vi "TEST - Current VIs Parents Ref.vi"(8 "error in (no error)":errorcluster) -> (0 "error out":errorcluster, 2 "pass":bool)   [LabVIEW 2009]
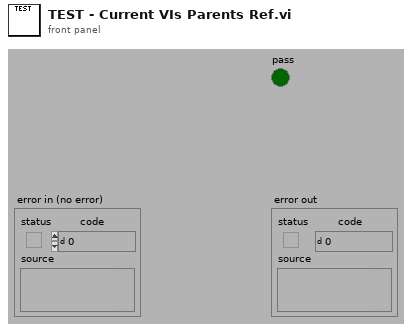
[diagram p1: front panel]
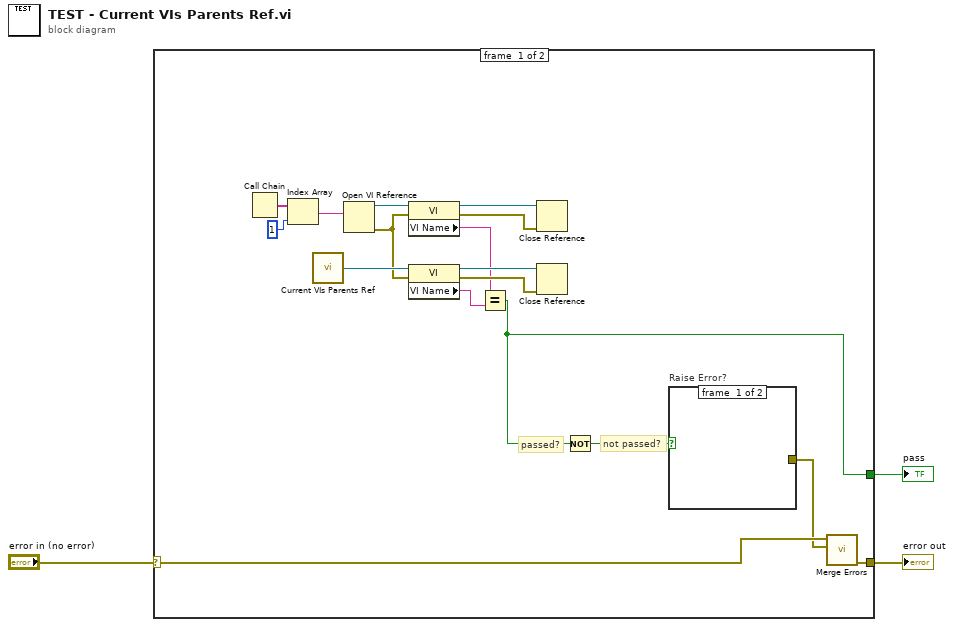
[diagram p0: block diagram]
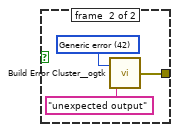
[diagram p2: hidden frame]
diagram:
  n1 = case shown="No Error" "error in (no error)" {
    selector: "error in (no error)" -> [w20 w24]
    tunnel: [w4 _] -> w3
    tunnel: [w19 w24] -> w1
    frame #0 {
      # "not passed?"
      # "passed?"
      n2 = Call Chain() -> (call chain=w16:string[])
      n3 = Index Array(array=w16, index=1 ("Index")) -> (element=w14:string)
      n4 = call "Current VIs Parents Ref.vi"() -> ("Calling VI's reference"=w8:refnum<vi>)  [unwired: 2 in]
      n5 = Open VI Reference(vi path=w14) -> (vi reference=w13:refnum<vi>, error out=w5:errorcluster)  [unwired: 5 in]
      n6 = property class="VI"(reference=w13, error in=w5) -> (reference out=w12:refnum<vi>, error out=w11:errorcluster, "VI Name"=w6:string)
      n7 = property class="VI"(reference=w8, error in=w5) -> (reference out=w9:refnum<vi>, error out=w10:errorcluster, "VI Name"=w7:string)
      n8 = Equal?(x=w6, y=w7) -> (x = y?=w4:bool)
      n9 = Close Reference(reference=w12, error in (no error)=w11) -> ()  [unwired: 1 out]
      n10 = Close Reference(reference=w9, error in (no error)=w10) -> ()  [unwired: 1 out]
      n11 = Not(x=w4) -> (.not. x?=w17:bool)
      n12 = case "Raise Error?" shown="True" w17 {
        tunnel: [_ w21] -> w18
        frame #0 {
        }
        frame #1 {
          w22 = 42 items=["No error", "Argument error", "Memory is full", "Out of zone", "End of file", "File already open", "Generic file I/O error", "File not found", "File permission error", "Disk is full", "Duplicate path", "Too many files open", "System feature not enabled", "Resource file not found", "Cannot add resource", "Resource not found", "Image not found", "Image memory error", "Pen does not exist", "Config type invalid", "Config token not found", "Config parse error", "Config memory error", "Bad external code format", "Bad external code offset", "External code not present", "Null window", "Destroy window error", "Null menu", "Print aborted", "Bad print record", "Print driver error", "Windows error during printing", "Memory error during printing", "Print dialog error", "Generic print error", "Invalid device refnum", "Device not found", "Device parameter error", "Device unit error", "Cannot open device", "Device call aborted", "Generic error", "Cancelled by user", "Object ID too low", "Object ID too high", "Object not in heap", "Unknown heap", "Unknown object (invalid DefProc)", "Unknown object (DefProc not in table)", "Message out of range", "Invalid (null) method", "Unknown message", "Manager call not supported", "Bad address", "Network operation in progress", "Network operation timed out", "Connection is busy", "Network attribute not supported", "Network error", "Address in use", "System out of memory", "Connection aborted", "Connection refused", "Not connected", "Already connected", "Connection closed", "Initialization error (interapplication manager)", "Bad occurrence", "Wait on unbound occurrence handler", "Occurrence queue overflow", "Datalog type conflict", "Unused", "Unrecognized type (interapplication manager)", "Memory corrupt", "Failed to make temporary DLL", "Old CIN version", "Drag socket not found", "Failed to load drop-object", "Failed to register OLE object", "Failed to release OLE object", "Format specifier type mismatch", "Unknown format specifier", "Too few format specifiers", "Too many format specifiers", "Scan failed", "Newer CIN version", "Error converting to variant", "Runtime menu error", "Password tampered", "Variant attribute not found", "Incompatible variant data type", "Event data is not available", "Event Store is not present", "Occurrence is not found", "Event Queue is not created", "Event info is not available", "Refnum passed is NULL", "Error retrieving Class GUID", "Error retrieving CoClass GUID", "Error retrieving TypeLib GUID.", "Bad built application magic bytes.", "Specific driver is different from the specific driver associated with the Logical Name.", "There is no session opened to the class driver.", "Max Error", "MAX - Error with config objects", "MAX - Error loading configuration", "MAX - Group not supported"]
          n13 = call <userlib>:"Build Error Cluster__ogtk.vi"("String to Prepend to source (\"\")"="unexpected output" ("String to Prepend to source (\"\")"), "code"=w22) -> ("error out"=w21:errorcluster)
        }
      }
      n14 = call <vilib>:"Merge Errors.vi"("error in 2 (no error)"=w18, "error in 1 (no error)"=w20) -> ("error out"=w19:errorcluster)  [unwired: 5 in]
    }
    frame #1 {
    }
  }
  "pass" <- w3
  "error out" <- w1
